vi "xy graph utility.vi"(1 "redraw?":bool, 2 "y-wave columns":u8[](array[numeric]), 3 "show files":T1(array[cluster])=[{"String"="20120217.012", "Boolean"=TRUE, "begin"=15, "length"=10000, "y weight"=1.0}], 4 "XYGraph Refnum":refnum<vi>) -> ()   [LabVIEW 2020]
panel:
  out "filtered":T1(array[cluster])
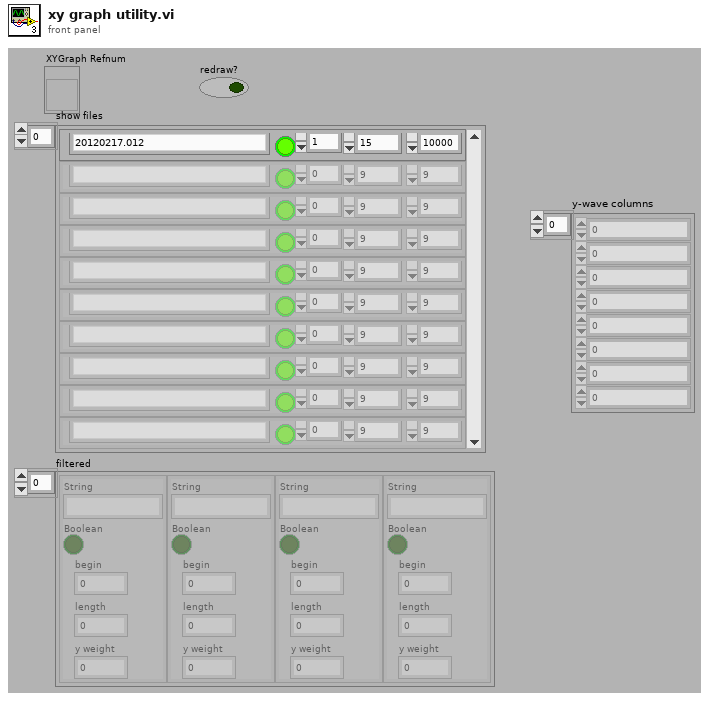
[diagram p1: front panel]
types:
  T1 = cluster{"String":string, "Boolean":bool, "begin":u32, "length":u32, "y weight":dbl}[]
  T2 = cluster{"String":string, "Boolean":bool, "begin":u32, "length":u32, "y weight":dbl}
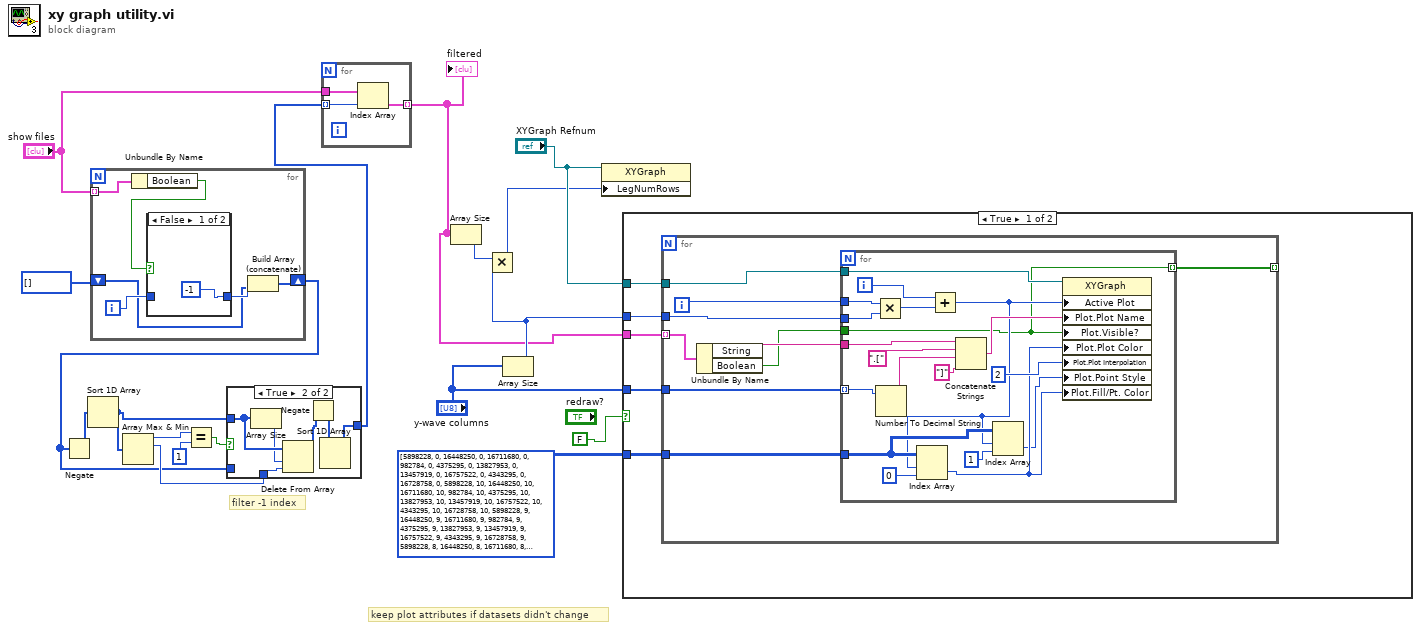
[diagram p0: block diagram]
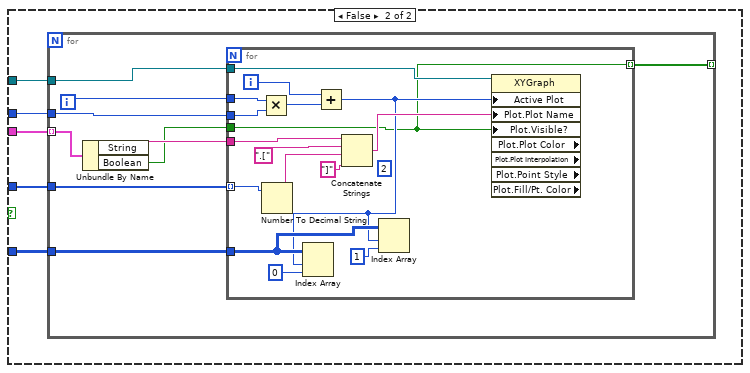
[diagram p2: hidden frame]
diagram:
  # "keep plot attributes if datasets didn't change"
  # "filter -1 index"
  n1 = for {
    tunnel: "show files" -> [w23] mode=indexing
    shift-right: [w19] -> w5
    shift-left: i32[] [] -> [w20]
    i -> [w21]
    n2 = Unbundle By Name(w23) -> ("Boolean"=w24:bool)
    n3 = case shown="False" w24 {
      tunnel: [-1 w26] -> w22
      tunnel: w21 -> [_ w26]
      frame False {
      }
      frame True {
      }
    }
    n4 = Build Array (concatenate)(w20, w22) -> (w19:i32[])
  }
  n5 = Negate(x=w5) -> (-x=w11:i32[])
  n6 = Sort 1D Array(array=w11) -> (sorted array=w10:i32[])
  n7 = Array Max & Min(array=w10) -> (max value=w6:i32, max index (indices)=w9:i32)  [unwired: 2 out]
  n8 = Equal?(x=w6, y=1) -> (x = y?=w8:bool)
  n9 = case shown="True" w8 {
    tunnel: w5 -> [w27 _]
    tunnel: [w27 w29] -> w2
    tunnel: w10 -> [_ w33]
    tunnel: w9 -> [_ w31]
    frame False {
    }
    frame True {
      n10 = Array Size(array=w33) -> (size(s)=w32:i32)
      n11 = Delete From Array(array=w33, length=w32, index=w31) -> (array with subset deleted=w30:i32[])  [unwired: 1 out]
      n12 = Negate(x=w30) -> (-x=w28:i32[])
      n13 = Sort 1D Array(array=w28) -> (sorted array=w29:i32[])
    }
  }
  n14 = for {
    tunnel: w2 -> [w36] mode=indexing
    tunnel: "show files" -> [w35]
    tunnel: [w34] -> w3 mode=indexing
    n15 = Index Array(array=w35, index=w36) -> (element=w34:T2)
  }
  "filtered" <- w3
  n16 = Array Size(array=w3) -> (size(s)=w15:i32)
  n17 = Array Size(array="y-wave columns") -> (size(s)=w14:i32)
  n18 = Multiply(x=w15, y=w14) -> (x*y=w13:i32)
  n19 = property class="XYGraph"(reference="XYGraph Refnum", "LegNumRows"=w13) -> ()  [unwired: 1 in, 2 out]
  n20 = case shown="True" FALSE {
    tunnel: "y-wave columns" -> [w41 w74]
    tunnel: u32[][] [[5898228, 0], [16448250, 0], [16711680, 0], [982784, 0], [4375295, 0], [13827953, 0], [13457919, 0], [16757522, 0], [4343295, 0], [16728758, 0], [5898228, 10], [16448250, 10], [16711680, 10], [982784, 10], [4375295, 10], [13827953, 10], [13457919, 10], [16757522, 10], [4343295, 10], [16728758, 10], [5898228, 9], [16448250, 9], [16711680, 9], [982784, 9], [4375295, 9], [13827953, 9], [13457919, 9], [16757522, 9], [4343295, 9], [16728758, 9], [5898228, 8], [16448250, 8], [16711680, 8], [982784, 8], [4375295, 8], [13827953, 8], [13457919, 8], [16757522, 8], [4343295, 8], [16728758, 8], [5898228, 7], [16448250, 7], [16711680, 7], [982784, 7], [4375295, 7], [13827953, 7], [13457919, 7], [16757522, 7], [4343295, 7], [16728758, 7], [5898228, 6], [16448250, 6], [16711680, 6], [982784, 6], [4375295, 6], [13827953, 6], [13457919, 6], [16757522, 6], [4343295, 6], [16728758, 6], [5898228, 5], [16448250, 5], [16711680, 5], [982784, 5], [4375295, 5], [13827953, 5], [13457919, 5], [16757522, 5], [4343295, 5], [16728758, 5], [5898228, 4], [16448250, 4], [16711680, 4], [982784, 4], [4375295, 4], [13827953, 4], [13457919, 4], [16757522, 4], [4343295, 4], [16728758, 4], [5898228, 3], [16448250, 3], [16711680, 3], [982784, 3], [4375295, 3], [13827953, 3], [13457919, 3], [16757522, 3], [4343295, 3], [16728758, 3], [5898228, 2], [16448250, 2], [16711680, 2], [982784, 2], [4375295, 2], [13827953, 2], [13457919, 2], [16757522, 2], [4343295, 2], [16728758, 2], [5898228, 1], [16448250, 1], [16711680, 1], [982784, 1], [4375295, 1], [13827953, 1], [13457919, 1], [16757522, 1], [4343295, 1], [16728758, 1]] ("Array") -> [w40 w73]
    tunnel: "XYGraph Refnum" -> [w39 w72]
    tunnel: w14 -> [w38 w71]
    tunnel: w3 -> [w37 w70]
    frame True {
      n21 = for {
        tunnel: w37 -> [w49] mode=indexing
        tunnel: w41 -> [w50]
        tunnel: w38 -> [w46]
        tunnel: w40 -> [w44]
        tunnel: w39 -> [w43]
        tunnel: [w42] -> _ mode=indexing
        i -> [w47]
        n22 = Unbundle By Name(w49) -> ("String"=w48:string, "Boolean"=w45:bool)
        n23 = for {
          tunnel: w50 -> [w68] mode=indexing
          tunnel: w48 -> [w69]
          tunnel: w47 -> [w64]
          tunnel: w46 -> [w63]
          tunnel: w45 -> [w51]
          tunnel: w44 -> [w57]
          tunnel: w43 -> [w56]
          tunnel: [w51] -> w42 mode=indexing
          i -> [w61]
          n24 = Multiply(x=w64, y=w63) -> (x*y=w62:i32)
          n25 = Number To Decimal String(number=w68) -> (decimal integer string=w66:string)  [unwired: 1 in]
          n26 = Add(x=w61, y=w62) -> (x+y=w52:i32)
          n27 = Index Array(array=w57, index (row)=w52, index (col)=0 ("disabled index (col)")) -> (element=w54:u32)
          n28 = Concatenate Strings(w69, ".[" ("string"), w66, "]" ("string")) -> (w60:string)
          n29 = Index Array(array=w57, index (row)=w52, index (col)=1 ("disabled index (col)")) -> (element=w53:u32)
          n30 = property class="XYGraph"(reference=w56, "Active Plot"=w52, "Plot.Plot Name"=w60, "Plot.Visible?"=w51, "Plot.Plot Color"=w54, "Plot.Plot Interpolation"=u8 2, "Plot.Point Style"=w53, "Plot.Fill/Pt. Color"=w54) -> ()  [unwired: 1 in, 2 out]
        }
      }
    }
    frame False {
      n31 = for {
        tunnel: w70 -> [w82] mode=indexing
        tunnel: w74 -> [w83]
        tunnel: w71 -> [w79]
        tunnel: w73 -> [w77]
        tunnel: w72 -> [w76]
        tunnel: [w75] -> _ mode=indexing
        i -> [w80]
        n32 = Unbundle By Name(w82) -> ("String"=w81:string, "Boolean"=w78:bool)
        n33 = for {
          tunnel: w83 -> [w98] mode=indexing
          tunnel: w81 -> [w99]
          tunnel: w80 -> [w94]
          tunnel: w79 -> [w93]
          tunnel: w78 -> [w84]
          tunnel: w77 -> [w87]
          tunnel: w76 -> [w86]
          tunnel: [w84] -> w75 mode=indexing
          i -> [w91]
          (unwired) u8 2 ("Plot.Plot Interpolation")
          n34 = Multiply(x=w94, y=w93) -> (x*y=w92:i32)
          n35 = Number To Decimal String(number=w98) -> (decimal integer string=w96:string)  [unwired: 1 in]
          n36 = Add(x=w91, y=w92) -> (x+y=w85:i32)
          n37 = Index Array(array=w87, index (row)=w85, index (col)=0 ("disabled index (col)")) -> ()  [unwired: 1 out]
          n38 = Concatenate Strings(w99, ".[" ("string"), w96, "]" ("string")) -> (w90:string)
          n39 = Index Array(array=w87, index (row)=w85, index (col)=1 ("disabled index (col)")) -> ()  [unwired: 1 out]
          n40 = property class="XYGraph" props=["Active Plot", "Plot", "Plot Name", "Plot", "Visible?", "Plot", "Plot Color", "Plot", "Plot Interpolation", "Plot", "Point Style", "Plot", "Fill/Pt. Color"](reference=w86, "Active Plot"=w85, "Plot.Plot Name"=w90, "Plot.Visible?"=w84) -> ()  [unwired: 1 in, 6 out]
        }
      }
    }
  }
